vi "P2018 TB INCAR_Run Manual.vi"(7 "Comunicaciones":T7={"Flujo_1"="ASRL6::INSTR", "Brk1"=FALSE, "Flujo_2"="ASRL6::INSTR", "Brk2"=FALSE, "Flujo_3"="ASRL6::INSTR", "Brk3"=FALSE, "Flujo_4"="ASRL6::INSTR", "Brk4"=FALSE, "Eurothe"="ASRL6::INSTR", "Eurot"=FALSE, "Balanza"="ASRL6::INSTR", "Bal"=FALSE, "eValPos"="ASRL6::INSTR", "eVal"=FALSE, "flowbus"="ASRL6::INSTR", "fb"=FALSE}, 8 "error in (no error)":errorcluster) -> (0 "error out":errorcluster)   [LabVIEW 2013]
uses:
  Controles/P2022 Datos Control.ctl
  Controles/P2018 Com Control.ctl
  modbusEurotherm P116_485/P2018 Eurotherm Control.ctl
  modbusEurotherm P116_485/4xP116.ctl
  Controles/P2018 Bronkhorst Control.ctl
  serialBronkhorst/_s_TablaBronkhorst.ctl
  Controles/P2018 DisbalTB Control.ctl
  Controles/P2018 Arduino Control.ctl
  Controles/Data Type.ctl
  Display/Display_Command Control.ctl
  Controles/P2018 runManual Control.ctl
  File/File_Module Control.ctl
  Timing/Timing_Module Control.ctl
  modbusEurotherm P116_485/Eurotherm_Hardware_Module Control.ctl
  serialTermobDisbal/Multicard III_Hardware_Module Control.ctl
  Controles/Change Control.ctl
  P2022 TB INCAR GLOBALES.vi
panel:
  out "FLOWBUS_MassFlows":T1={"Dispositivos"=[["3", "NO", "M0000013", "Air", "10", "ln/mn", "0", "0"], ["4", "NO", "M0000014", "Air", "10", "ln/mn", "0", "0"], ["5", "NO", "M0000015", "Air", "10", "ln/mn", "0", "0"], ["6", "NO", "M0000016", "Air", "10", "ln/mn", "0", "0"], ["7", "NO", "M0000017", "Air", "10", "ln/mn", "0", "0"], ["8", "NO", "M0000018", "Air", "10", "ln/mn", "0", "0"]], "NuevosSP"=[["0", "NO", "M0000013", "Air", "1", "ln/mn", "0", "0"], ["0", "NO", "M0000014", "Air", "1", "ln/mn", "0", "0"], ["0", "NO", "M0000015", "Air", "1", "ln/mn", "0", "0"], ["0", "NO", "M0000016", "Air", "1", "ln/mn", "0", "0"], ["0", "NO", "M0000017", "Air", "1", "ln/mn", "0", "0"], ["0", "NO", "M0000018", "Air", "1", "ln/mn", "0", "0"]], "Nodes"=4, "Delay(s)"=0.075}
  out "Time Elapsed":bool
  out "ARDUINO":T3
  out "TIEMPO (m)":dbl
  out "DISBAL":T4 caption="tarjetaPresion"
  out "Fecha":string caption="asd"
  out "SERIAL_MassFlows":T1={"Dispositivos"=[["3", "NO", "M0000013", "Air", "10", "ln/mn", "0", "0"], ["4", "NO", "M0000014", "Air", "10", "ln/mn", "0", "0"], ["5", "NO", "M0000015", "Air", "10", "ln/mn", "0", "0"], ["6", "NO", "M0000016", "Air", "10", "ln/mn", "0", "0"], ["7", "NO", "M0000017", "Air", "10", "ln/mn", "0", "0"], ["8", "NO", "M0000018", "Air", "10", "ln/mn", "0", "0"]], "NuevosSP"=[["0", "NO", "M0000013", "Air", "1", "ln/mn", "0", "0"], ["0", "NO", "M0000014", "Air", "1", "ln/mn", "0", "0"], ["0", "NO", "M0000015", "Air", "1", "ln/mn", "0", "0"], ["0", "NO", "M0000016", "Air", "1", "ln/mn", "0", "0"], ["0", "NO", "M0000017", "Air", "1", "ln/mn", "0", "0"], ["0", "NO", "M0000018", "Air", "1", "ln/mn", "0", "0"]], "Nodes"=4, "Delay(s)"=0.075}
  out "EURO_P116":T5
  out "Time":string caption="asd"
  out "Date":string caption="asd"
  out "ERRORES_T":i32=5 caption="Elapsed Time (s)"
  out "errorT":bool
  out "DATOS":T8 {"fFSET4" format="%.2g"; "fFSET3" format="%.2g"; "fFSET2" format="%.2g"; "fFSET1" format="%.2g"; "fFLUJO4" format="%.2g"; "fFLUJO2" format="%.2g"; "fFLUJO1" format="%.2g"; "fFLUJO3" format="%.2g"; "T_EXTRA" format="%.2g"; "TSET_EXTRA" format="%.2g"; "T_CINTA" format="%.2g"; "TSET_CINTA" format="%.2g"; "sFSET4" format="%.2g"; "POSICION" format="%.2g"; "TEMP_SUP" format="%.2g"; "TSET_SUP" format="%.2g"; "PESO_TB" format="%.2g"; "TEMP_TB" format="%.2g"; "TEMP_INF" format="%.2g"; "sFSET3" format="%.2g"; "sFSET2" format="%.2g"; "sFSET1" format="%.2g"; "V_VAPOR" format="%.2g"; "sFLUJO4" format="%.2g"; "sFLUJO2" format="%.2g"; "sFLUJO1" format="%.2g"; "TSET_INF" format="%.2g"; "TIEMPO" format="%.2g"; "sFLUJO3" format="%.2g"}
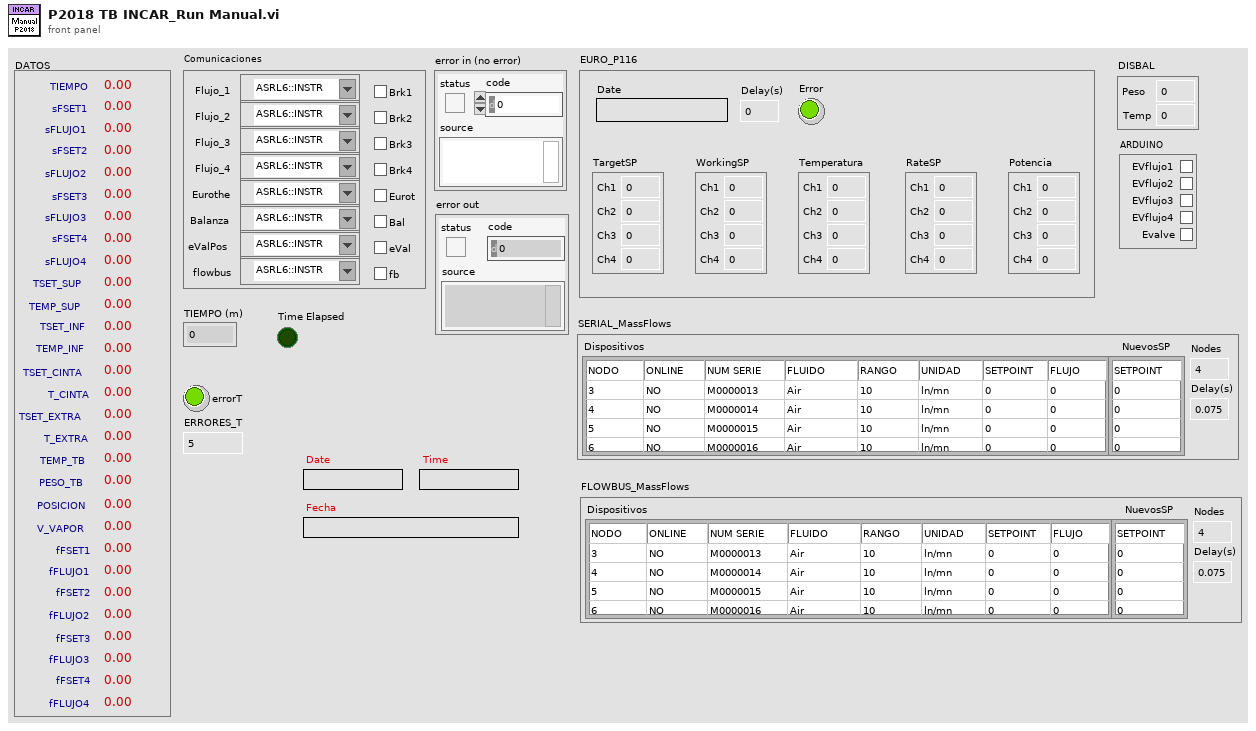
[diagram p1: front panel]
types:
  T1 = typedef "P2018 Bronkhorst Control.ctl" = cluster{"Dispositivos":T2, "NuevosSP":string[][], "Nodes":u32, "Delay(s)":dbl}
  T2 = typedef "_s_TablaBronkhorst.ctl" = string[][]
  T3 = typedef "P2018 Arduino Control.ctl" = cluster{"EVflujo1":bool, "EVflujo2":bool, "EVflujo3":bool, "EVflujo4":bool, "Evalve":bool}
  T4 = typedef "P2018 DisbalTB Control.ctl" = cluster{"Peso":dbl, "Temp":dbl}
  T5 = typedef "P2018 Eurotherm Control.ctl" = cluster{"TargetSP":T6, "WorkingSP":T6, "Temperatura":T6, "Error":bool, "Date":string, "Delay(s)":dbl, "RateSP":T6, "Potencia":T6}
  T6 = typedef "4xP116.ctl" = cluster{"Ch1":dbl, "Ch2":dbl, "Ch3":dbl, "Ch4":dbl}
  T7 = typedef "P2018 Com Control.ctl" = cluster{"Flujo_1":refnum<visa-resource-name>, "Brk1":bool, "Flujo_2":refnum<visa-resource-name>, "Brk2":bool, "Flujo_3":refnum<visa-resource-name>, "Brk3":bool, "Flujo_4":refnum<visa-resource-name>, "Brk4":bool, "Eurothe":refnum<visa-resource-name>, "Eurot":bool, "Balanza":refnum<visa-resource-name>, "Bal":bool, "eValPos":refnum<visa-resource-name>, "eVal":bool, "flowbus":refnum<visa-resource-name>, "fb":bool}
  T8 = typedef "P2022 Datos Control.ctl" = cluster{"TIEMPO":dbl, "sFSET1":dbl, "sFLUJO1":dbl, "sFSET2":dbl, "sFLUJO2":dbl, "sFSET3":dbl, "sFLUJO3":dbl, "sFSET4":dbl, "sFLUJO4":dbl, "TSET_SUP":dbl, "TEMP_SUP":dbl, "TSET_INF":dbl, "TEMP_INF":dbl, "TSET_CINTA":dbl, "T_CINTA":dbl, "TSET_EXTRA":dbl, "T_EXTRA":dbl, "TEMP_TB":dbl, "PESO_TB":dbl, "POSICION":dbl, "V_VAPOR":dbl, "fFSET1":dbl, "fFLUJO1":dbl, "fFSET2":dbl, "fFLUJO2":dbl, "fFSET3":dbl, "fFLUJO3":dbl, "fFSET4":dbl, "fFLUJO4":dbl}
  T9 = typedef "Data Type.ctl" = enum16{"Init FP", "En/Dis FP Ctls", "Update FP", "Upd Status", "Upd Seq"}
  T10 = typedef "Display_Command Control.ctl" = enum16{"Initialize", "Generate Event", "Shutdown"}
  T11 = typedef "P2018 runManual Control.ctl" = enum16{"INICIALIZAR", "READ BRONKHORST", "READ EUROTHERM", "READ DISBAL", "READ ARDUINO", "ESPERAR", "CAMBIOS", "GUARDAR", "FINALIZAR"}
  T12 = typedef "Timing_Module Control.ctl" = enum16{"Initialize Time", "Check Time"}
  T13 = typedef "File_Module Control.ctl" = enum16{"Initialize", "Save Head", "Save Data", "Shutdown"}
  T14 = typedef "Eurotherm_Hardware_Module Control.ctl" = enum16{"Initialize", "Write SP", "Read SP+PV", "Write Rate", "Set P", "Set I", "Set D", "Shutdown"}
  T15 = typedef "Multicard III_Hardware_Module Control.ctl" = enum16{"Initialize", "Cero", "Span", "Read ugr", "Read mgr", "Read A/D", "Read T", "Number readings", "Thermocouple type", "Status", "Shutdown"}
  T16 = typedef "Change Control.ctl" = enum16{"Default", "Continue", "Change Flows", "Change Valves", "Change Temp"}
  T17 = typedef "_f_TablaBronkhorst.ctl" = string[][]
  T18 = enum16{"Add 1", "Add 2", "Add 10", "Add 11", "Add 12", "Add 13"}[]
  T19 = cluster{"processVal":dbl, "targetSP":dbl, "workingSP":dbl, "workingOut":dbl}
  T20 = cluster{"[0]":dbl, "[1]":dbl, "[2]":dbl, "[3]":dbl}
  T21 = typedef "P2019 SetpointsFlows.ctl" = cluster{"SP1":dbl, "SP2":dbl, "SP3":dbl, "SP4":dbl}
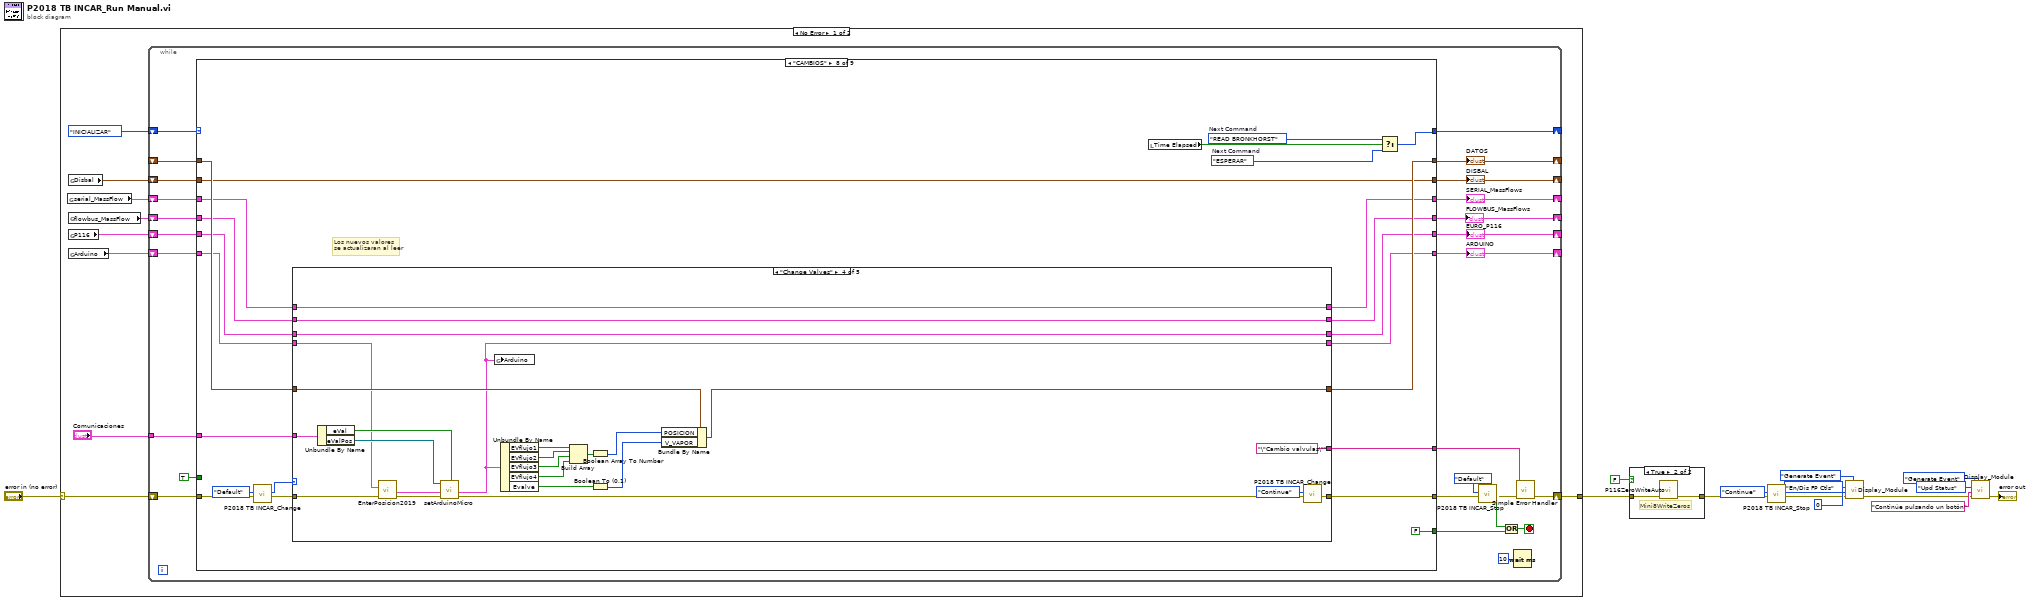
[diagram p0: block diagram]
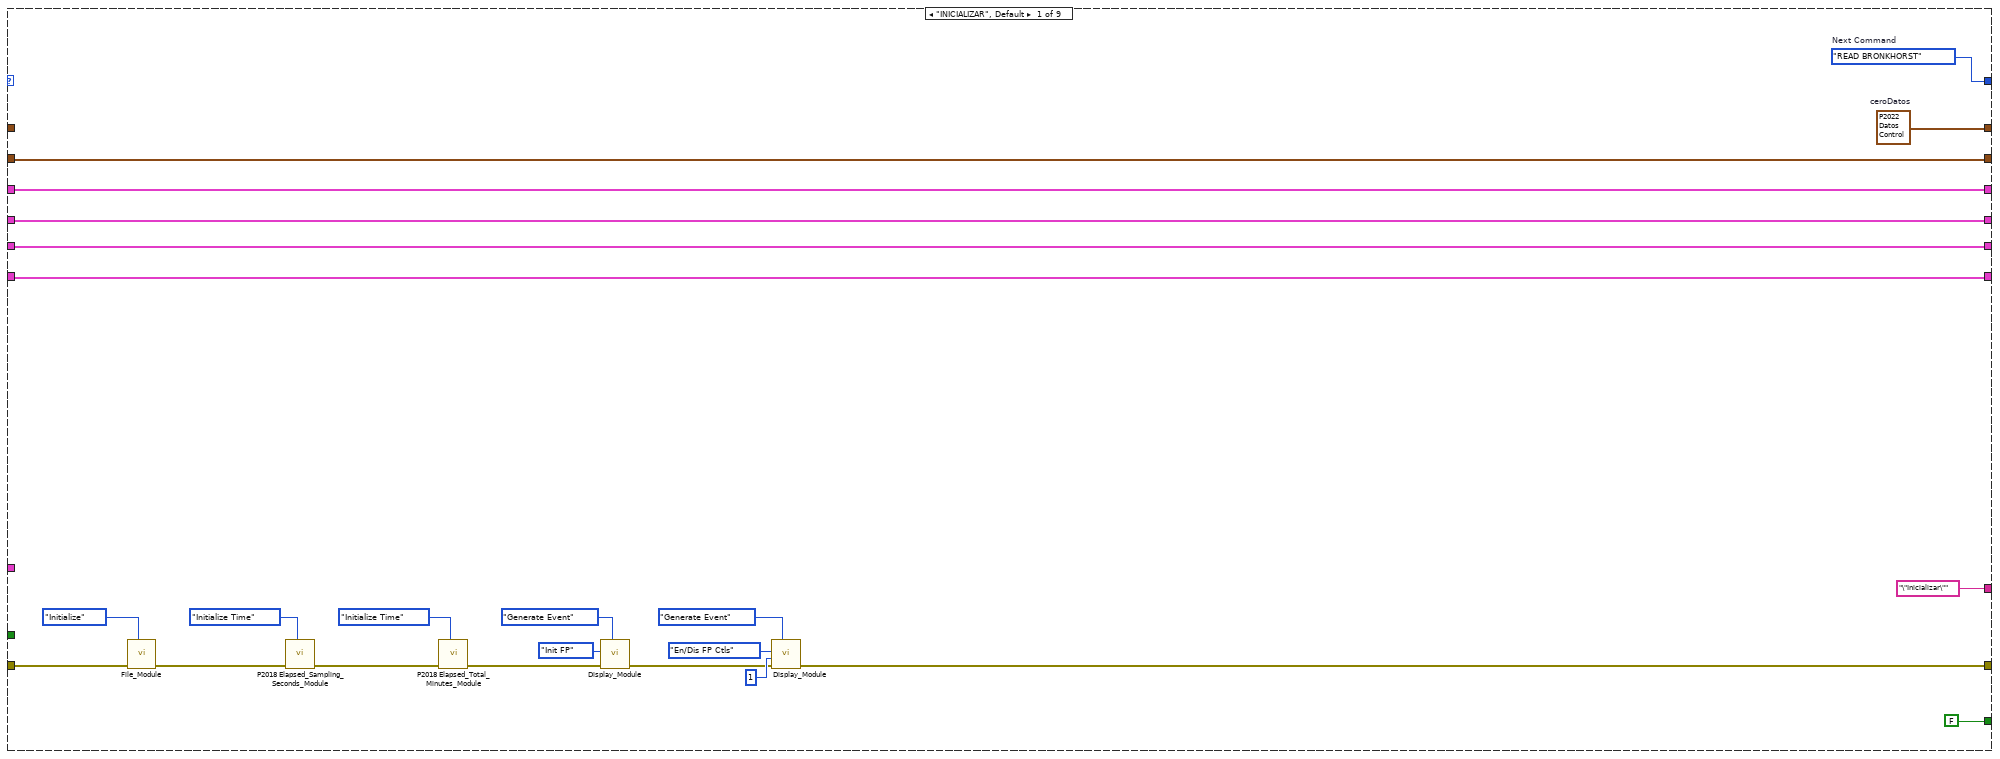
[diagram p3: hidden frame]
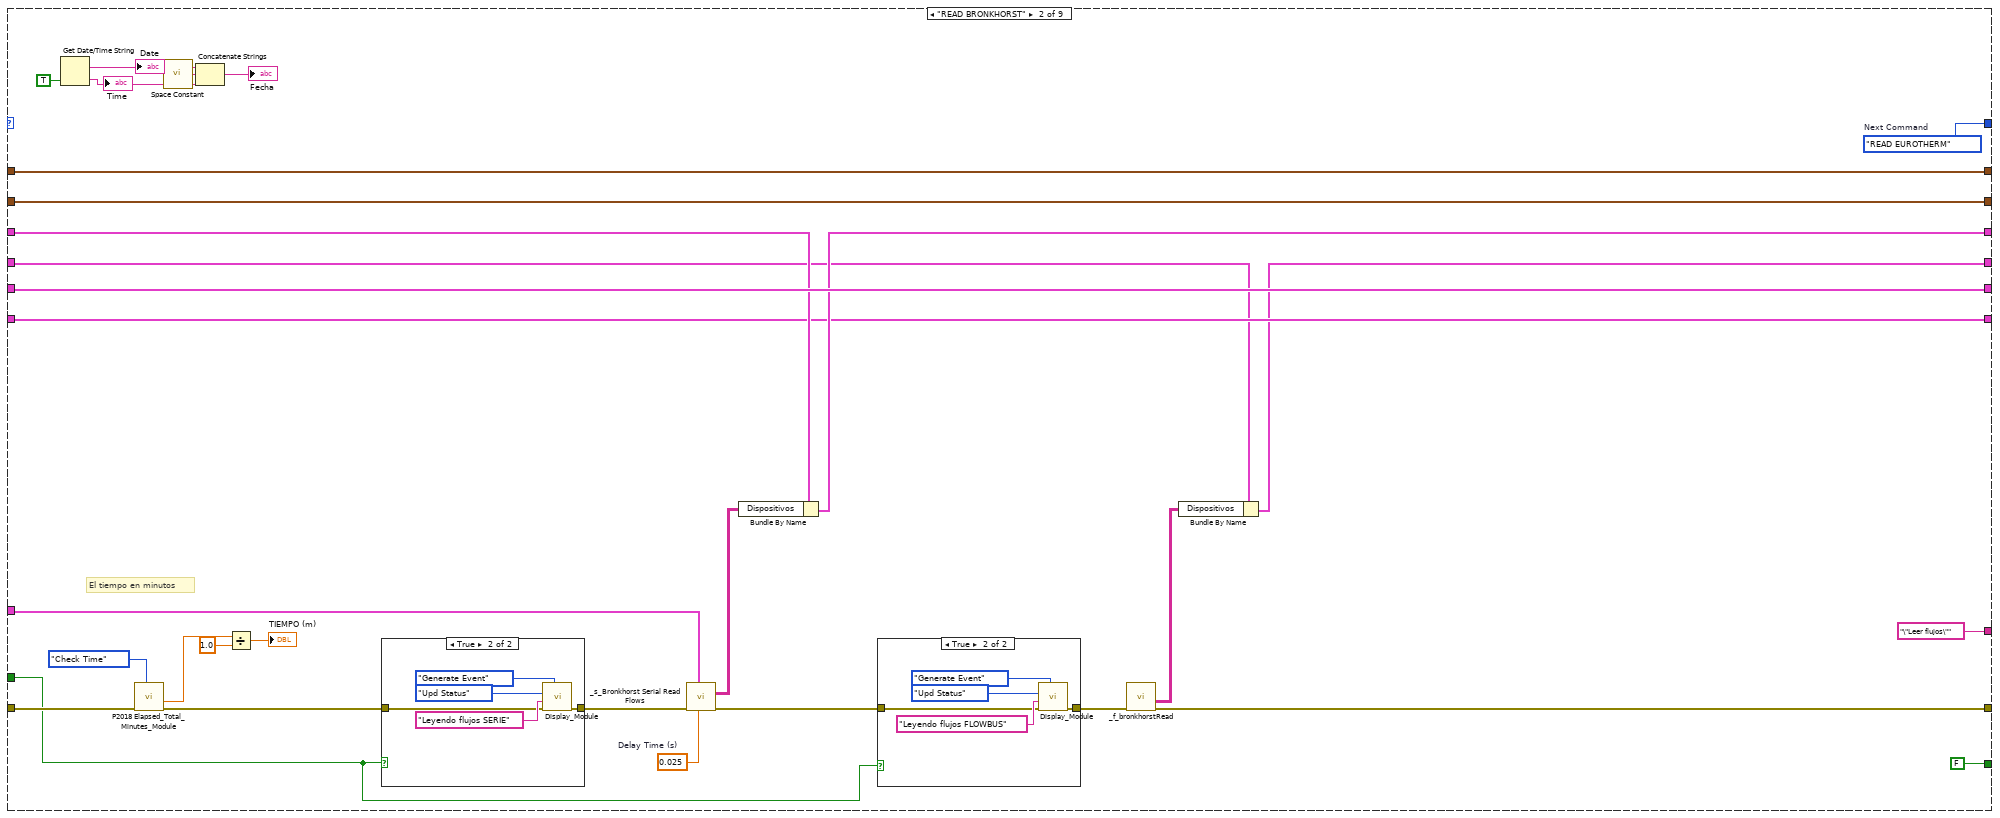
[diagram p4: hidden frame]
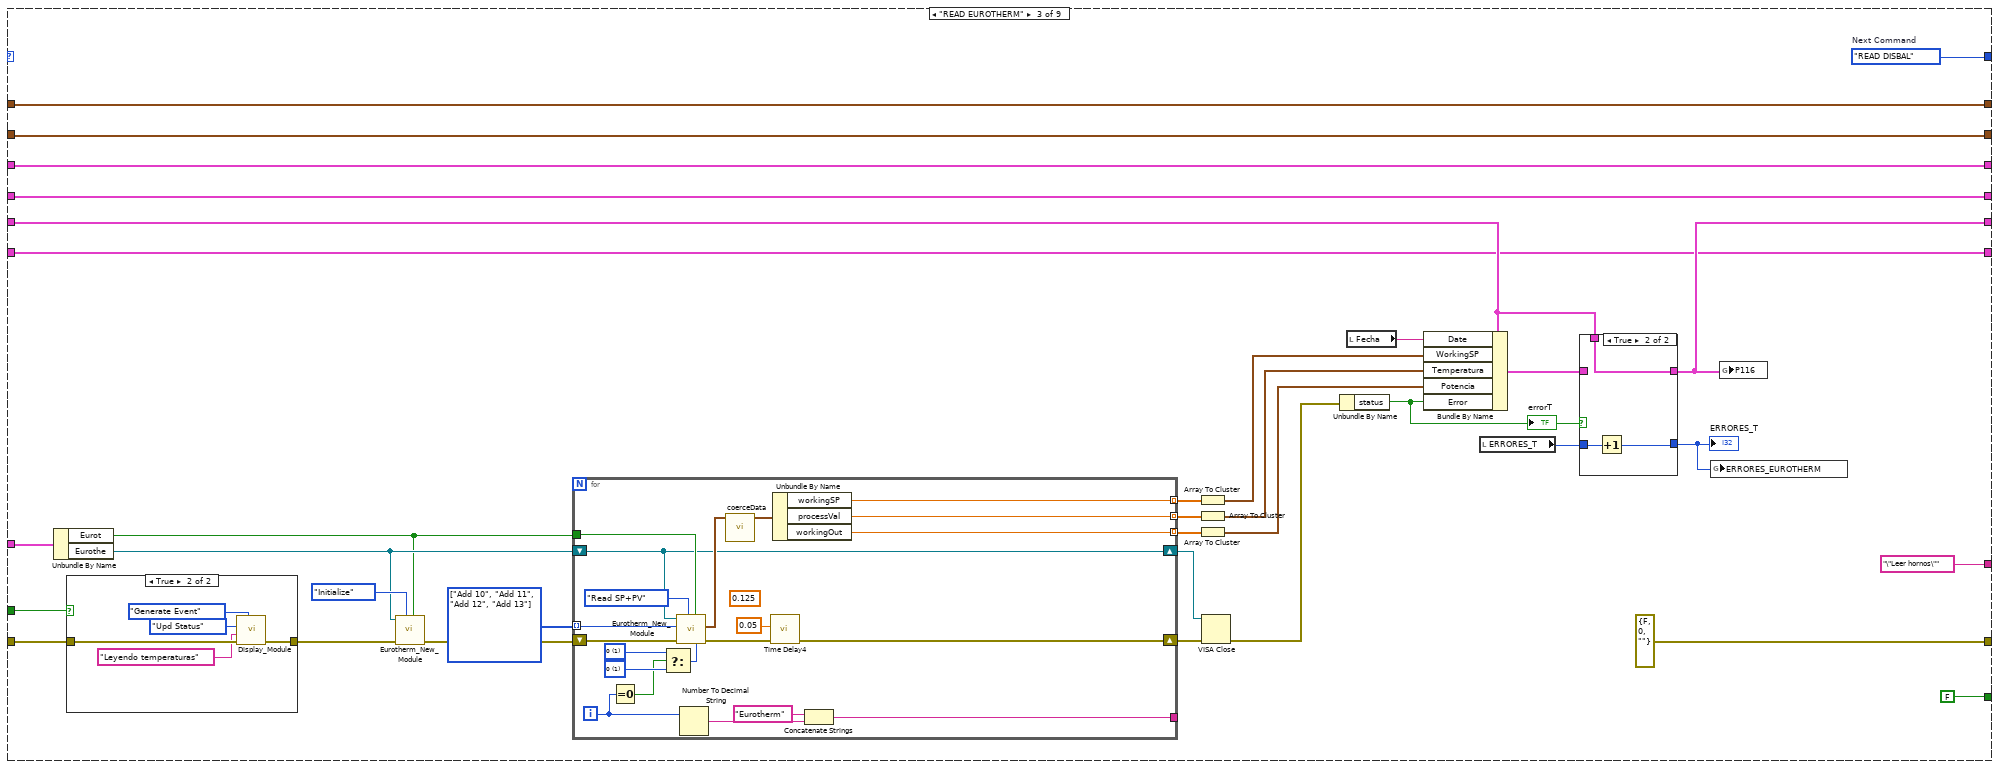
[diagram p7: hidden frame]
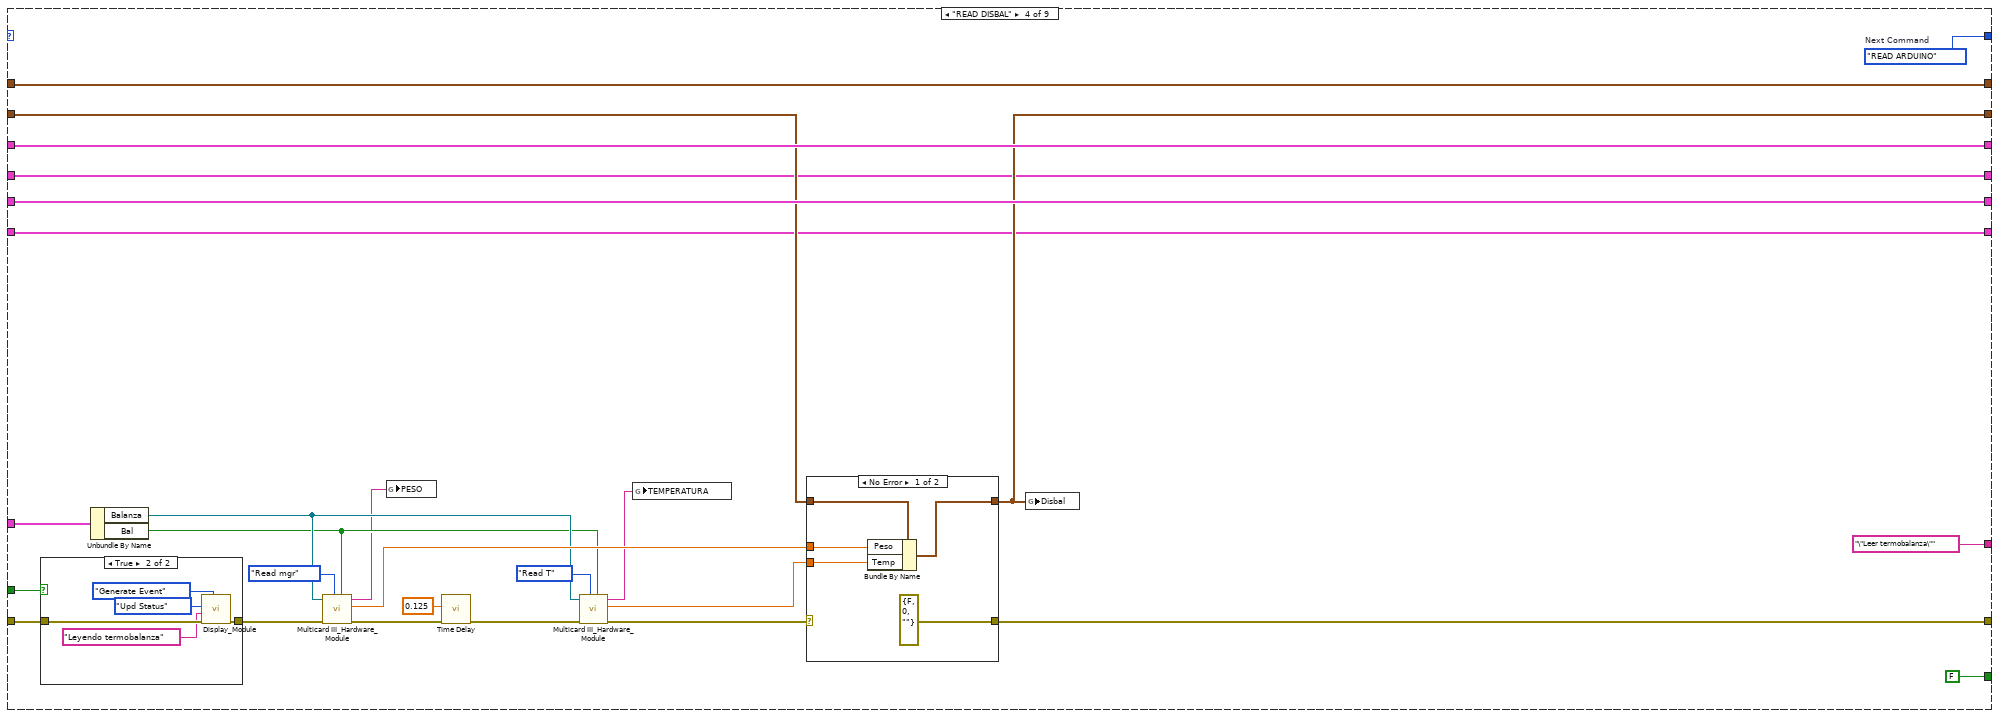
[diagram p10: hidden frame]
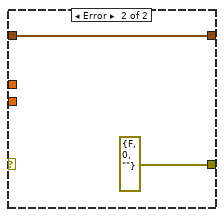
[diagram p12: hidden frame]
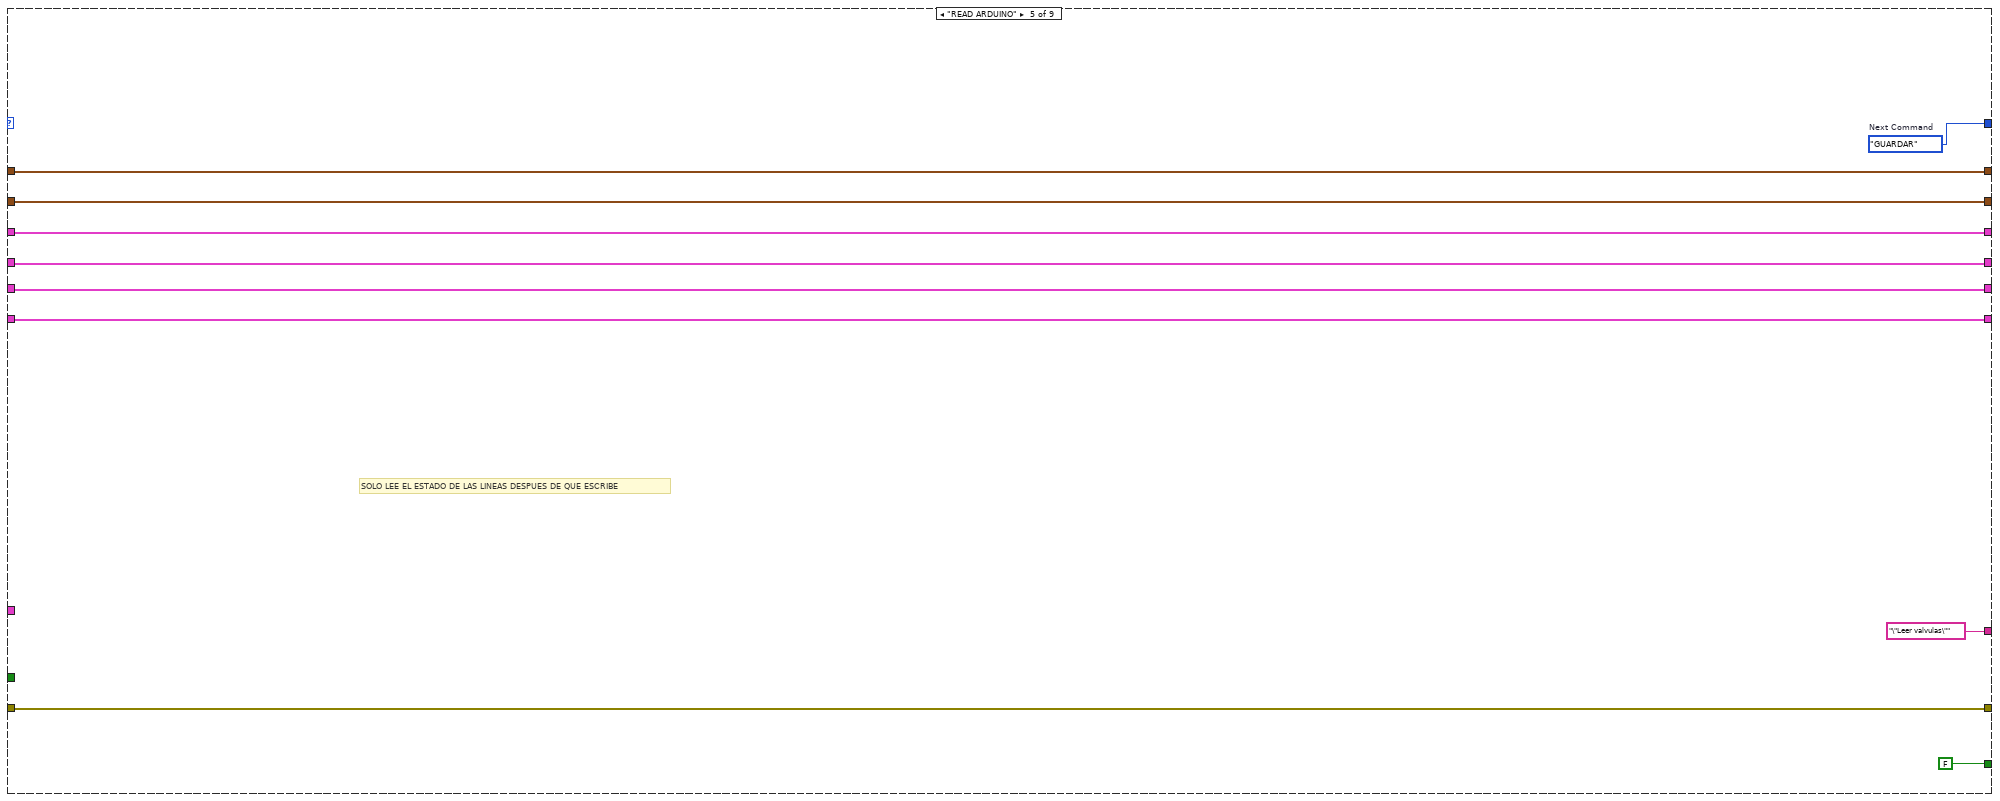
[diagram p13: hidden frame]
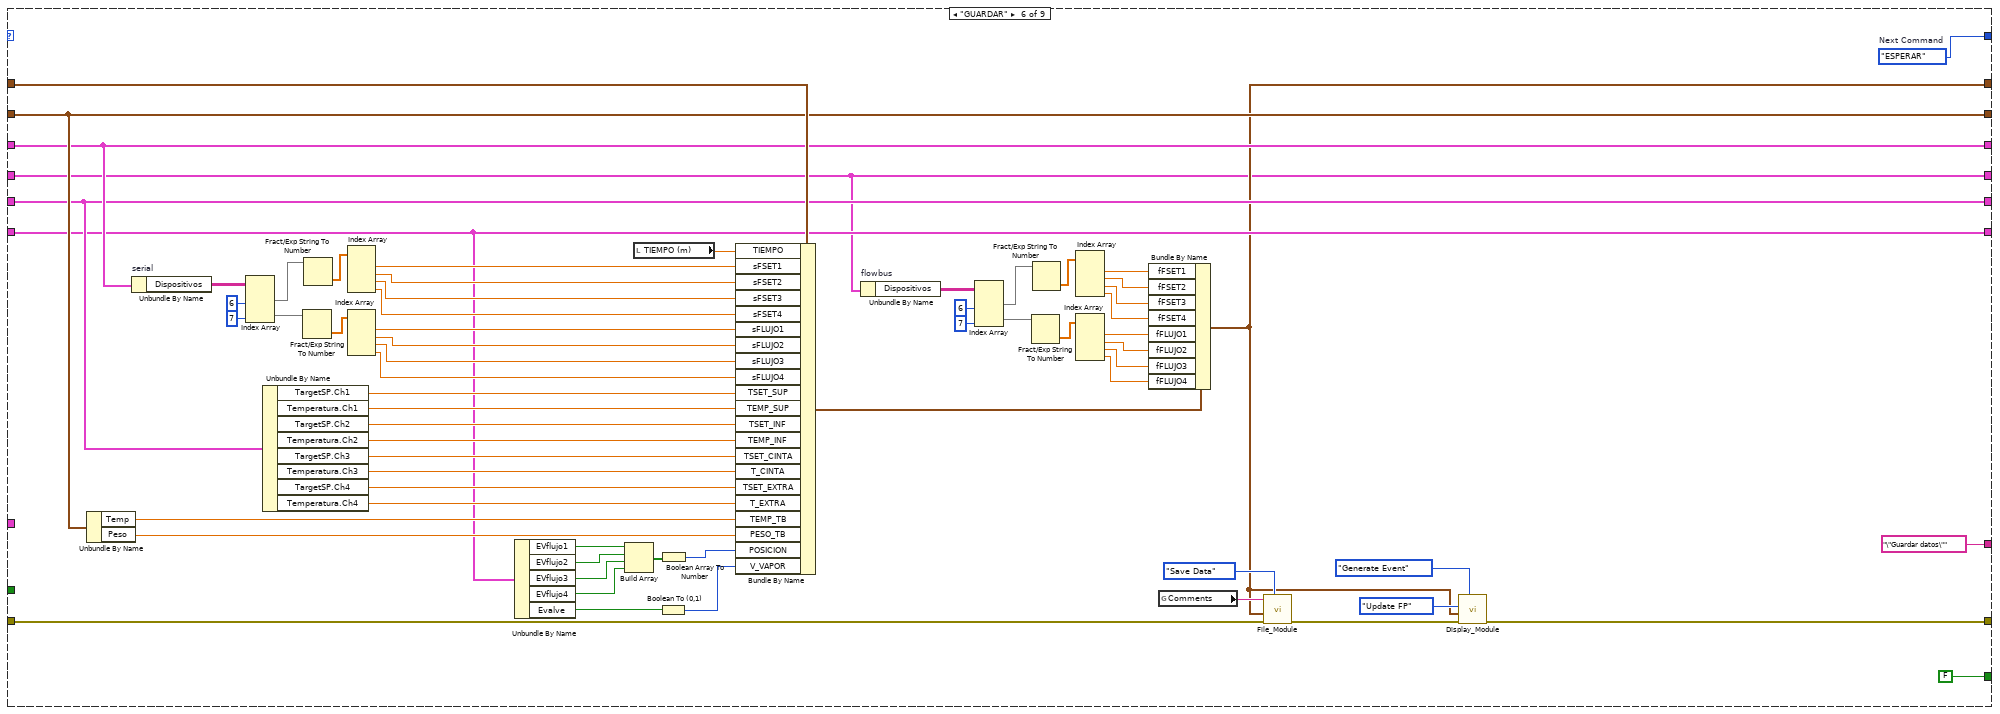
[diagram p14: hidden frame]
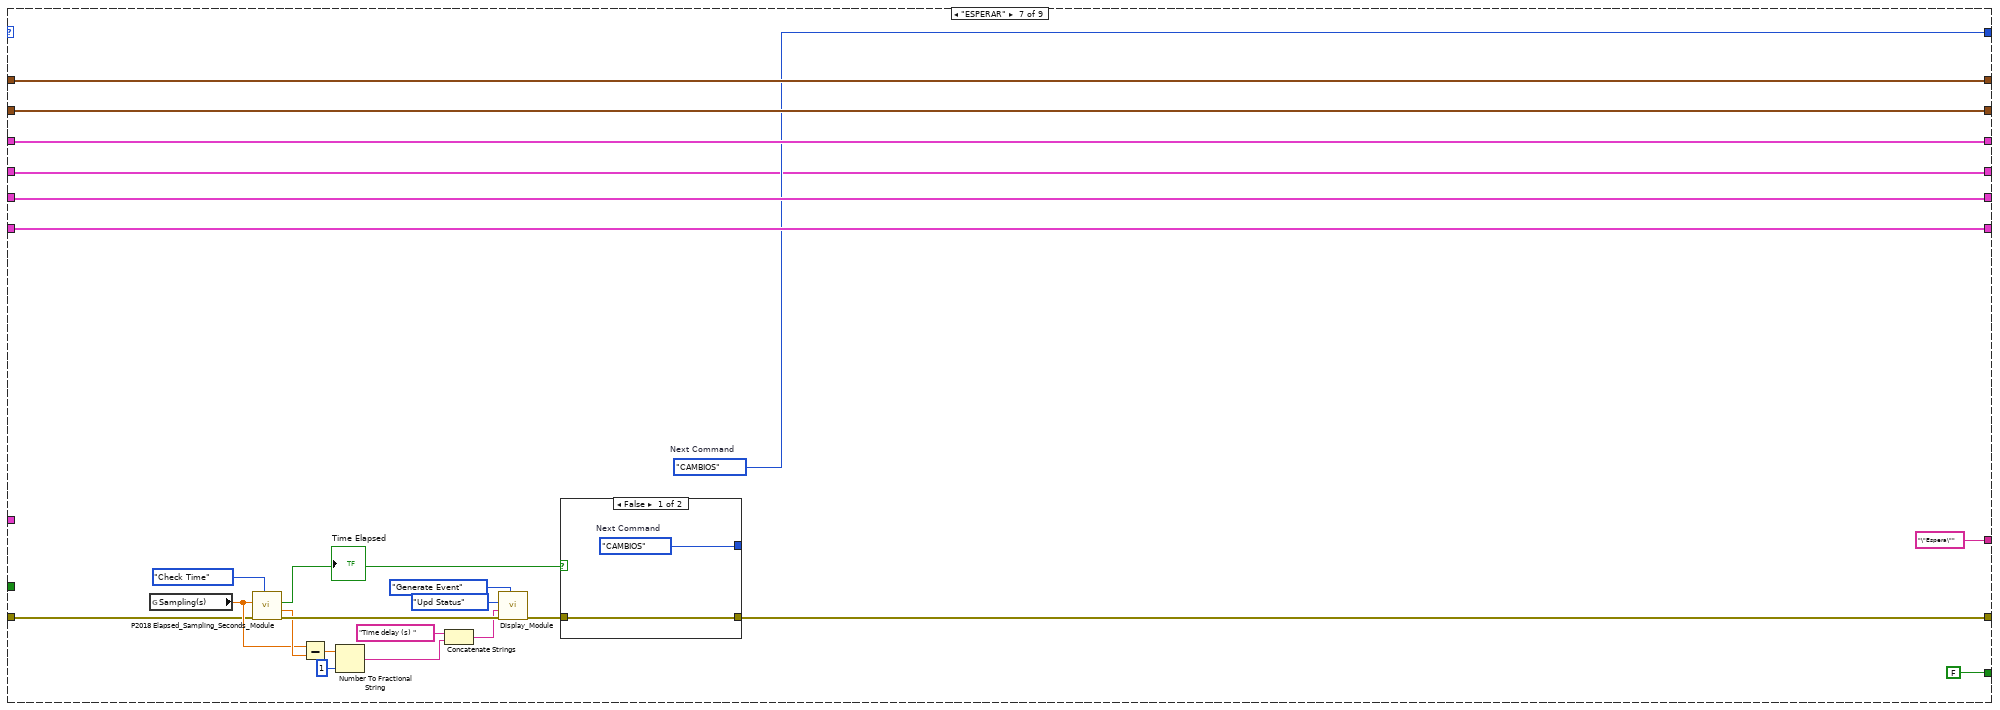
[diagram p15: hidden frame]
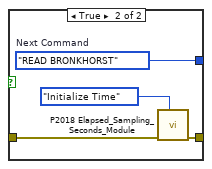
[diagram p16: hidden frame]
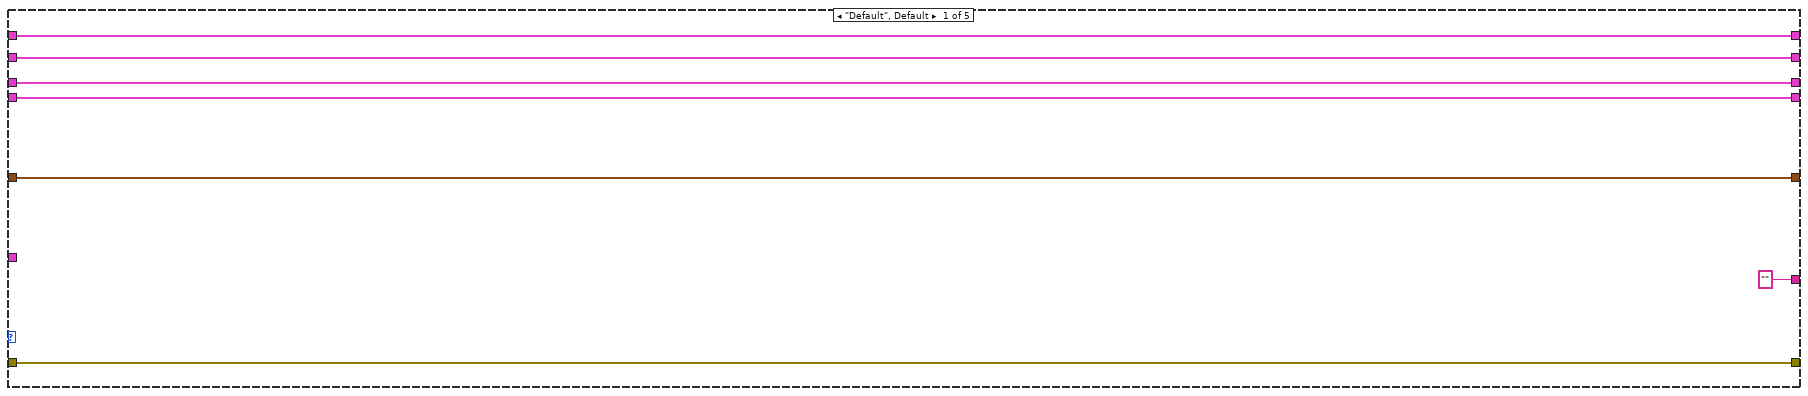
[diagram p17: hidden frame]
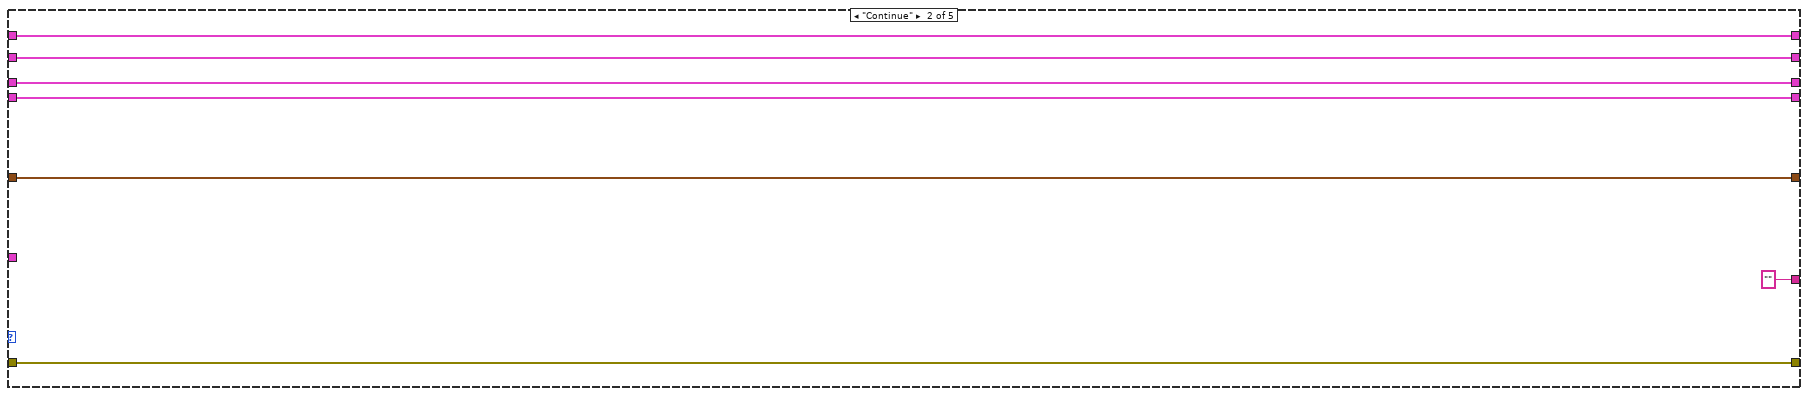
[diagram p18: hidden frame]
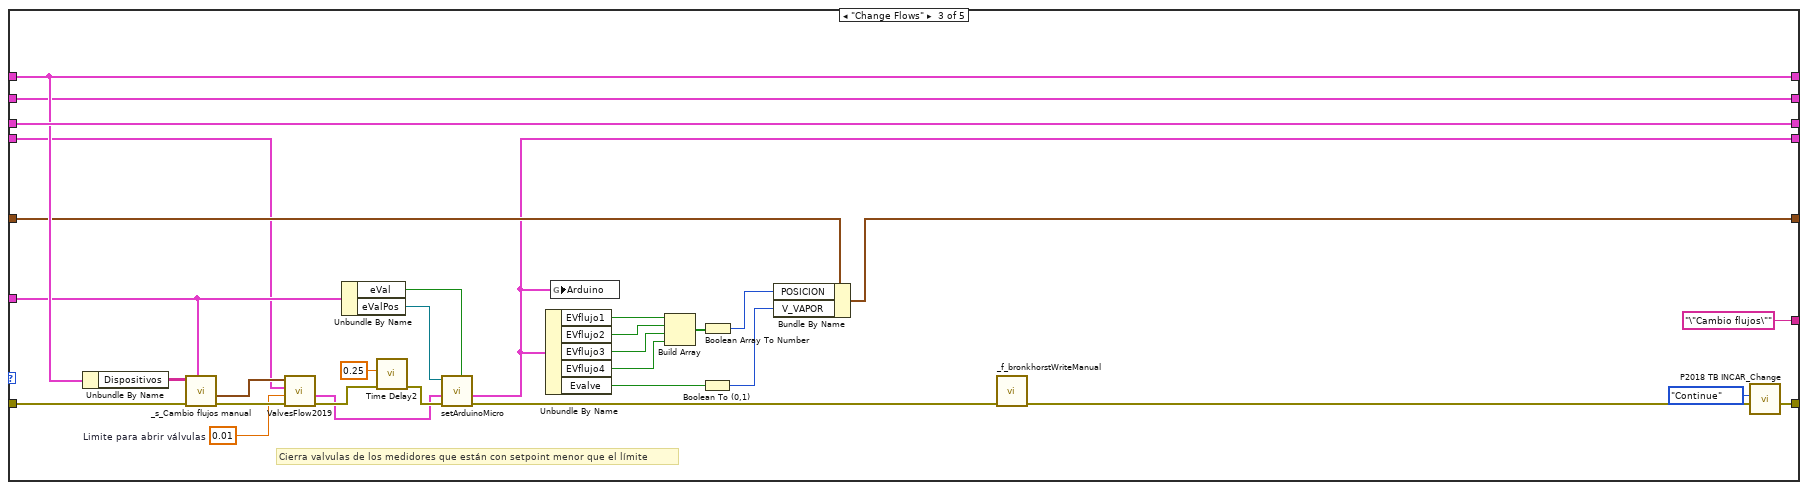
[diagram p19: hidden frame]
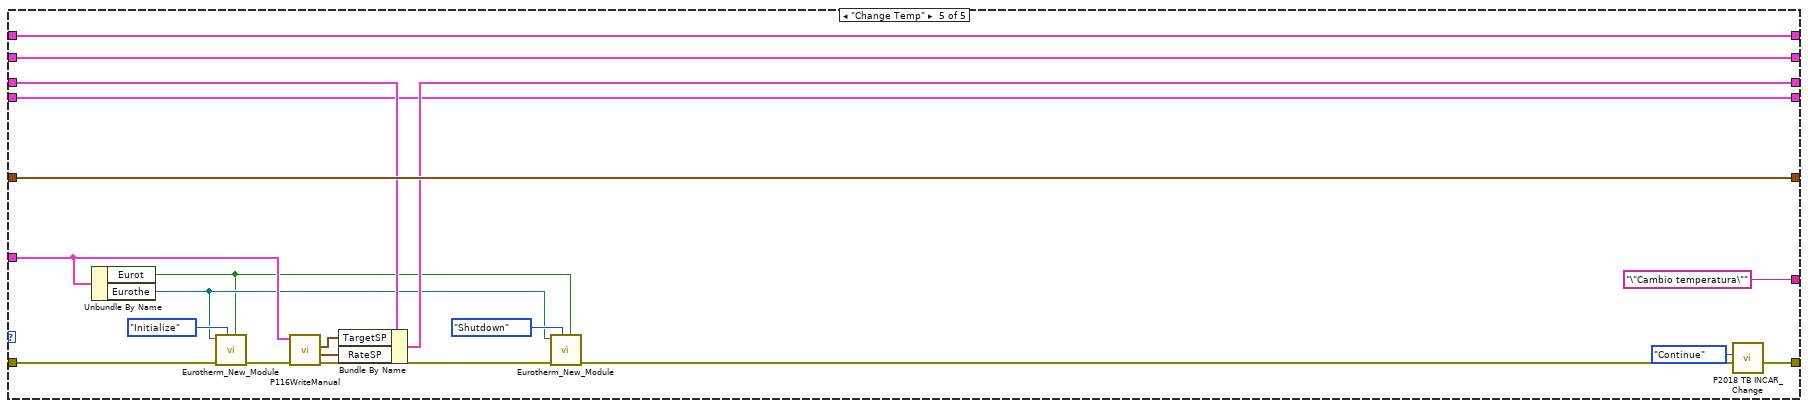
[diagram p20: hidden frame]
diagram:
  n1 = case shown="No Error" "error in (no error)" {
    selector: "error in (no error)" -> [w23 w453]
    tunnel: [w22 w453] -> w2
    frame No Error {
      n2 = global read "P2022 TB INCAR GLOBALES.vi" "serial_MassFlow"() -> (w18:T1)
      n3 = global read "P2022 TB INCAR GLOBALES.vi" "Disbal"() -> (w17:T4)
      n4 = global read "P2022 TB INCAR GLOBALES.vi" "flowbus_MassFlow"() -> (w15:T1)
      n5 = global read "P2022 TB INCAR GLOBALES.vi" "P116"() -> (w19:T5)
      n6 = global read "P2022 TB INCAR GLOBALES.vi" "Arduino"() -> (w16:T3)
      n7 = while {
        shift-right: [w42] -> _
        shift-left: P2018_runManual_Control."INICIALIZAR" ("Command") -> [w45]
        shift-right: [w36] -> w22
        shift-left: w23 -> [w46]
        shift-right: [w41] -> _
        shift-left: _ -> [w40]
        tunnel: "Comunicaciones" -> [w38]
        shift-right: [w30] -> _
        shift-left: w18 -> [w34]
        shift-right: [w32] -> _
        shift-left: w19 -> [w33]
        shift-right: [w29] -> _
        shift-left: w17 -> [w31]
        shift-right: [w27] -> _
        shift-left: w16 -> [w28]
        shift-right: [w24] -> _
        shift-left: w15 -> [w25]
        stop <- w48 stop-if-true
        n8 = case shown="\"CAMBIOS\"" w45 {
          tunnel: [FALSE FALSE FALSE FALSE FALSE FALSE FALSE FALSE TRUE] -> w47
          tunnel: w46 -> [w71 w91 w148 w207 w228 w298 w306 w350 w451]
          tunnel: [w69 w79 errorcluster {"status"=FALSE, "code"=0, "source"=""} ("error out") w204 w228 w292 w319 w347 w451] -> w44
          tunnel: [w65 w102 w147 w205 w230 w290 w300 w332 w449] -> w42
          tunnel: [w70 w82 w133 w190 w229 w233 w318 w344 w450] -> w41
          tunnel: w40 -> [_ w82 w133 w190 w229 w289 w318 w345 w450]
          tunnel: w38 -> [_ w92 w146 w202 _ _ _ w343 _]
          tunnel: ["\"Inicializar\"" ("error source (\" \")") "\"Leer flujos\"" ("error source (\" \")") "\"Leer hornos\"" ("error source (\" \")") "\"Leer termobalanza\"" ("error source (\" \")") "\"Leer valvulas\"" ("error source (\" \")") "\"Guardar datos\"" ("error source (\" \")") "\"Espera\"" ("error source (\" \")") w342 "\"Finalizar\"" ("error source (\" \")")] -> w35
          tunnel: [w53 w85 w121 w191 w226 w285 w303 w337 w446] -> w30
          tunnel: w34 -> [w53 w86 w121 w191 w226 w285 w303 w338 w446]
          tunnel: [w54 w98 w120 w192 w225 w277 w304 w339 w447] -> w32
          tunnel: w33 -> [w54 w98 w130 w192 w225 w277 w304 w340 w447]
          tunnel: w31 -> [w52 w83 w119 w189 w224 w288 w302 w341 w445]
          tunnel: [w52 w83 w119 w188 w224 w288 w302 w341 w445] -> w29
          tunnel: [w51 w81 w118 w187 w223 w252 w301 w335 w444] -> w27
          tunnel: w28 -> [w51 w81 w118 w187 w223 w252 w301 w336 w444]
          tunnel: TRUE -> [_ w73 w117 w185 _ _ _ _ _]
          tunnel: w25 -> [w50 w77 w116 w184 w222 w232 w299 w330 w443]
          tunnel: [w50 w76 w116 w184 w222 w232 w299 w329 w443] -> w24
          frame "INICIALIZAR", Default {
            w65 = P2018_runManual_Control."READ BRONKHORST"  # Next Command
            w70 = T8 {"TIEMPO"=0.0, "sFSET1"=0.0, "sFLUJO1"=0.0, "sFSET2"=0.0, "sFLUJO2"=0.0, "sFSET3"=0.0, "sFLUJO3"=0.0, "sFSET4"=0.0, "sFLUJO4"=0.0, "TSET_SUP"=0.0, "TEMP_SUP"=0.0, "TSET_INF"=0.0, "TEMP_INF"=0.0, "TSET_CINTA"=0.0, "T_CINTA"=0.0, "TSET_EXTRA"=0.0, "T_EXTRA"=0.0, "TEMP_TB"=0.0, "PESO_TB"=0.0, "POSICION"=0.0, "V_VAPOR"=0.0, "fFSET1"=0.0, "fFLUJO1"=0.0, "fFSET2"=0.0, "fFLUJO2"=0.0, "fFSET3"=0.0, "fFLUJO3"=0.0, "fFSET4"=0.0, "fFLUJO4"=0.0}  # ceroDatos
            n9 = call "File_Module.vi"("Command"=File_Module_Control."Initialize", "error in (no error)"=w71) -> ("error out"=w58:errorcluster)  [unwired: 8 in, 1 out]
            n10 = call "P2018 Elapsed_Sampling_Seconds_Module.vi"("Command"=Timing_Module_Control."Initialize Time", "error in (no error)"=w58) -> ("error out"=w60:errorcluster)  [unwired: 7 in, 2 out]
            n11 = call "P2018 Elapsed_Total_Minutes_Module.vi"("Command"=Timing_Module_Control."Initialize Time", "error in (no error)"=w60) -> ("error out"=w61:errorcluster)  [unwired: 7 in, 2 out]
            n12 = call "Display_Module.vi"("Command"=Display_Command_Control."Generate Event", "error in (no error)"=w61, "Data Type"=Data_Type."Init FP") -> ("error out"=w62:errorcluster)  [unwired: 8 in]
            n13 = call "Display_Module.vi"("Command"=Display_Command_Control."Generate Event", "error in (no error)"=w62, "Data"=1, "Data Type"=Data_Type."En/Dis FP Ctls") -> ("error out"=w69:errorcluster)  [unwired: 7 in]
          }
          frame "READ BRONKHORST" {
            w80 = 0.025  # Delay Time (s)
            w102 = P2018_runManual_Control."READ EUROTHERM"  # Next Command
            # "El tiempo en minutos"
            n14 = Get Date/Time String(want seconds? (F)=TRUE) -> (date string=w97:string, time string=w96:string)  [unwired: 2 in]
            "Time" <- w96
            "Date" <- w97
            n15 = call "P2018 Elapsed_Total_Minutes_Module.vi"("Command"=Timing_Module_Control."Check Time", "error in (no error)"=w91) -> ("error out"=w88:errorcluster, "Elapsed Out"=w90:dbl)  [unwired: 7 in, 1 out]
            n16 = call <vilib>:"Space Constant.vi"() -> ("String"=w94:string)
            n17 = Concatenate Strings(w97, w94, w96) -> (→"Fecha":string)
            n18 = Divide(x=w90, y=1.0) -> (x/y=→"TIEMPO (m)":dbl)
            n19 = case shown="True" w73 {
              tunnel: [w110 w112] -> w89
              tunnel: w88 -> [w110 w111]
              frame False {
              }
              frame True {
                n20 = call "Display_Module.vi"("Command"=Display_Command_Control."Generate Event", "error in (no error)"=w111, "Data"="Leyendo flujos SERIE", "Data Type"=Data_Type."Upd Status") -> ("error out"=w112:errorcluster)  [unwired: 7 in]
              }
            }
            n21 = call "_s_Bronkhorst Serial Read Flows.vi"("Delay Time (s)"=w80, "Comunicaciones"=w92, "error in (no error)"=w89) -> ("error out"=w75:errorcluster, "Dispositivos"=w84:T2)  [unwired: 7 in]
            n22 = Bundle By Name(cluster=w86, "Dispositivos"=w84) -> (w85:T1)
            n23 = case shown="True" w73 {
              tunnel: [w104 w106] -> w74
              tunnel: w75 -> [w104 w105]
              frame False {
              }
              frame True {
                n24 = call "Display_Module.vi"("Command"=Display_Command_Control."Generate Event", "error in (no error)"=w105, "Data"="Leyendo flujos FLOWBUS", "Data Type"=Data_Type."Upd Status") -> ("error out"=w106:errorcluster)  [unwired: 7 in]
              }
            }
            n25 = call "_f_bronkhorstRead.vi"("error in (no error)"=w74) -> ("error out"=w79:errorcluster, "Dispositivos"=w78:T17)  [unwired: 9 in]
            n26 = Bundle By Name(cluster=w77, "Dispositivos"=w78) -> (w76:T1)
          }
          frame "READ EUROTHERM" {
            w142 = T18 [enum."Add 10", enum."Add 11", enum."Add 12", enum."Add 13"] items=["Add 1", "Add 2", "Add 10", "Add 11", "Add 12", "Add 13"]
            w147 = P2018_runManual_Control."READ DISBAL"  # Next Command
            n27 = Unbundle By Name(w146) -> ("Eurot"=w139:bool, "Eurothe"=w140:refnum<visa-resource-name>)
            n28 = case shown="True" w117 {
              tunnel: w148 -> [w150 w153]
              tunnel: [w150 w151] -> w141
              frame False {
              }
              frame True {
                n29 = call "Display_Module.vi"("Command"=Display_Command_Control."Generate Event", "error in (no error)"=w153, "Data"="Leyendo temperaturas", "Data Type"=Data_Type."Upd Status") -> ("error out"=w151:errorcluster)  [unwired: 7 in]
              }
            }
            n30 = call "Eurotherm_New_Module.vi"("Eurotherm (T:Enable)"=w139, "Command"=Eurotherm_Hardware_Module_Control."Initialize", "error in (no error)"=w141, "VISA resource name"=w140) -> ("error out"=w143:errorcluster)  [unwired: 6 in, 1 out]
            n31 = for {
              tunnel: w142 -> [w175] mode=indexing
              tunnel: [w167] -> w136 mode=indexing
              tunnel: [w166] -> w135 mode=indexing
              shift-right: [w163] -> w137
              shift-left: w143 -> [w177]
              tunnel: w139 -> [w174]
              tunnel: [w179] -> _
              tunnel: [w165] -> w134 mode=indexing
              shift-right: [w164] -> w138
              shift-left: w140 -> [w164]
              i -> [w173]
              (unwired) 0.125 ("Delay Time (s)")
              w171 = u16 1 items=["0"=1, "1"=10, "2"=100] ("Decimales")
              w172 = u16 1 items=["0"=1, "1"=10, "2"=100] ("Decimales")
              n32 = Equal To 0?(x=w173) -> (x = 0?=w170:bool)
              n33 = Select(t=w172, s=w170, f=w171) -> (s? t:f=w169:u16)
              n34 = call "Eurotherm_New_Module.vi"("Decimales"=w169, "Eurotherm (T:Enable)"=w174, "Command"=Eurotherm_Hardware_Module_Control."Read SP+PV", "error in (no error)"=w177, "Address"=w175, "VISA resource name"=w164) -> ("error out"=w176:errorcluster, "Eurotherm"=w168:T19)  [unwired: 4 in]
              n35 = Number To Decimal String(number=w173) -> (decimal integer string=w180:string)  [unwired: 1 in]
              n36 = call "coerceData.vi"("Eurotherm"=w168) -> ("Eurotherm 2"=w161:T19)  [unwired: 10 in]
              n37 = call "Time Delay4"("error in (no error)"=w176, "Delay Time (s)"=0.05) -> ("error out"=w163:errorcluster)  [unwired: 9 in]
              n38 = Unbundle By Name(w161) -> ("workingSP"=w167:dbl, "processVal"=w166:dbl, "workingOut"=w165:dbl)
              n39 = Concatenate Strings("Eurotherm" ("error source (\" \")"), w180) -> (w179:string)
            }
            n40 = Array To Cluster(array=w136) -> (cluster=w128:T20)
            n41 = Array To Cluster(array=w135) -> (cluster=w127:T20)
            n42 = Array To Cluster(array=w134) -> (cluster=w126:T20)
            n43 = VISA Close(VISA resource name=w138, error in (no error)=w137) -> (error out=w125:errorcluster)
            n44 = Unbundle By Name(w125) -> ("status"=w132:bool)
            "errorT" <- w132
            n45 = local read "Fecha"() -> (w129:string)
            n46 = Bundle By Name(cluster=w130, "Date"=w129, "WorkingSP"=w128, "Temperatura"=w127, "Potencia"=w126, "Error"=w132) -> (w131:T5)
            n47 = local read "ERRORES_T"() -> (w123:i32)
            n48 = case shown="True" w132 {
              tunnel: w131 -> [w157 _]
              tunnel: [w157 w160] -> w120
              tunnel: w130 -> [_ w160]
              tunnel: w123 -> [w156 w159]
              tunnel: [w156 w158] -> w122
              frame False {
              }
              frame True {
                n49 = Increment(x=w159) -> (x+1=w158:i32)
              }
            }
            "ERRORES_T" <- w122
            n50 = global write "P2022 TB INCAR GLOBALES.vi" "ERRORES_EUROTHERM"(w122) -> ()
            n51 = global write "P2022 TB INCAR GLOBALES.vi" "P116"(w120) -> ()
          }
          frame "READ DISBAL" {
            w205 = P2018_runManual_Control."READ ARDUINO"  # Next Command
            n52 = case shown="True" w185 {
              tunnel: w207 -> [w209 w212]
              tunnel: [w209 w211] -> w206
              frame False {
              }
              frame True {
                n53 = call "Display_Module.vi"("Command"=Display_Command_Control."Generate Event", "error in (no error)"=w212, "Data"="Leyendo termobalanza", "Data Type"=Data_Type."Upd Status") -> ("error out"=w211:errorcluster)  [unwired: 7 in]
              }
            }
            n54 = Unbundle By Name(w202) -> ("Balanza"=w195:refnum<visa-resource-name>, "Bal"=w186:bool)
            n55 = call "Multicard III_Hardware_Module.vi"("Multicard (T:Enable)"=w186, "Command"=Multicard_III_Hardware_Module_Control."Read mgr", "error in (no error)"=w206, "VISA resource name"=w195) -> ("error out"=w197:errorcluster, "Output Value"=w203:dbl, "String"=w183:string)  [unwired: 4 in, 1 out]
            n56 = global write "P2022 TB INCAR GLOBALES.vi" "PESO"(w183) -> ()
            n57 = call "Time Delay"("error in (no error)"=w197, "Delay Time (s)"=0.125) -> ("error out"=w196:errorcluster)  [unwired: 9 in]
            n58 = call "Multicard III_Hardware_Module.vi"("Multicard (T:Enable)"=w186, "Command"=Multicard_III_Hardware_Module_Control."Read T", "error in (no error)"=w196, "VISA resource name"=w195) -> ("error out"=w199:errorcluster, "Output Value"=w198:dbl, "String"=w182:string)  [unwired: 4 in, 1 out]
            n59 = global write "P2022 TB INCAR GLOBALES.vi" "TEMPERATURA"(w182) -> ()
            n60 = case shown="No Error" w199 {
              tunnel: [errorcluster {"status"=FALSE, "code"=0, "source"=""} ("error out") errorcluster {"status"=FALSE, "code"=0, "source"=""} ("error out")] -> w204
              tunnel: w203 -> [w216 _]
              tunnel: w189 -> [w218 w220]
              tunnel: [w217 w220] -> w188
              tunnel: w198 -> [w215 _]
              frame No Error {
                n61 = Bundle By Name(cluster=w218, "Peso"=w216, "Temp"=w215) -> (w217:T4)
              }
              frame Error {
              }
            }
            n62 = global write "P2022 TB INCAR GLOBALES.vi" "Disbal"(w188) -> ()
          }
          frame "READ ARDUINO" {
            w230 = P2018_runManual_Control."GUARDAR"  # Next Command
            # "SOLO LEE EL ESTADO DE LAS LINEAS DESPUES DE QUE ESCRIBE"
          }
          frame "GUARDAR" {
            w290 = P2018_runManual_Control."ESPERAR"  # Next Command
            n63 = Unbundle By Name(w288) -> ("Temp"=w286:dbl, "Peso"=w287:dbl)
            n64 = Unbundle By Name "serial"(w285) -> ("Dispositivos"=w284:T2)
            n65 = Index Array(array=w284, index (col) #1=6 ("disabled index (col)"), index (col) #2=7 ("disabled index (col)")) -> (element #1=w265:string[], element #2=w266:string[])  [unwired: 2 in]
            n66 = Unbundle By Name(w277) -> ("TargetSP.Ch1"=w276:dbl, "Temperatura.Ch1"=w269:dbl, "TargetSP.Ch2"=w275:dbl, "Temperatura.Ch2"=w270:dbl, "TargetSP.Ch3"=w271:dbl, "Temperatura.Ch3"=w272:dbl, "TargetSP.Ch4"=w273:dbl, "Temperatura.Ch4"=w274:dbl)
            n67 = Fract/Exp String To Number(string=w266) -> (number=w281:dbl[])  [unwired: 3 in, 1 out]
            n68 = Fract/Exp String To Number(string=w265) -> (number=w264:dbl[])  [unwired: 3 in, 1 out]
            n69 = Index Array(array=w264) -> (element #1=w263:dbl, element #2=w262:dbl, element #3=w261:dbl, element #4=w260:dbl)  [unwired: 4 in]
            n70 = Index Array(array=w281) -> (element #1=w282:dbl, element #2=w280:dbl, element #3=w279:dbl, element #4=w278:dbl)  [unwired: 4 in]
            n71 = Unbundle By Name(w252) -> ("EVflujo1"=w257:bool, "EVflujo2"=w256:bool, "EVflujo3"=w255:bool, "EVflujo4"=w254:bool, "Evalve"=w258:bool)
            n72 = Build Array(w257, w256, w255, w254) -> (w253:bool[])
            n73 = local read "TIEMPO (m)"() -> (w268:dbl)
            n74 = Boolean To (0,1)(Boolean=w258) -> (0, 1=w251:i16)
            n75 = Boolean Array To Number(Boolean array=w253) -> (number=w250:u32)
            n76 = Bundle By Name(cluster=w289, "TIEMPO"=w268, "sFSET1"=w263, "sFSET2"=w262, "sFSET3"=w261, "sFSET4"=w260, "sFLUJO1"=w282, "sFLUJO2"=w280, "sFLUJO3"=w279, "sFLUJO4"=w278, "TSET_SUP"=w276, "TEMP_SUP"=w269, "TSET_INF"=w275, "TEMP_INF"=w270, "TSET_CINTA"=w271, "T_CINTA"=w272, "TSET_EXTRA"=w273, "T_EXTRA"=w274, "TEMP_TB"=w286, "PESO_TB"=w287, "POSICION"=w250, "V_VAPOR"=w251) -> (w234:T8)
            n77 = Unbundle By Name "flowbus"(w232) -> ("Dispositivos"=w243:T2)
            n78 = Index Array(array=w243, index (col) #1=6 ("disabled index (col)"), index (col) #2=7 ("disabled index (col)")) -> (element #1=w248:string[], element #2=w247:string[])  [unwired: 2 in]
            n79 = Fract/Exp String To Number(string=w247) -> (number=w245:dbl[])  [unwired: 3 in, 1 out]
            n80 = Fract/Exp String To Number(string=w248) -> (number=w249:dbl[])  [unwired: 3 in, 1 out]
            n81 = Index Array(array=w249) -> (element #1=w241:dbl, element #2=w240:dbl, element #3=w239:dbl, element #4=w238:dbl)  [unwired: 4 in]
            n82 = Index Array(array=w245) -> (element #1=w242:dbl, element #2=w237:dbl, element #3=w236:dbl, element #4=w235:dbl)  [unwired: 4 in]
            n83 = Bundle By Name(cluster=w234, "fFSET1"=w241, "fFSET2"=w240, "fFSET3"=w239, "fFSET4"=w238, "fFLUJO1"=w242, "fFLUJO2"=w237, "fFLUJO3"=w236, "fFLUJO4"=w235) -> (w233:T8)
            n84 = global read "P2022 TB INCAR GLOBALES.vi" "Comments"() -> (w259:string)
            n85 = call "File_Module.vi"("Command"=File_Module_Control."Save Data", "error in (no error)"=w298, "DATOS"=w233, "Comments"=w259) -> ("error out"=w293:errorcluster)  [unwired: 6 in, 1 out]
            n86 = call "Display_Module.vi"("Command"=Display_Command_Control."Generate Event", "error in (no error)"=w293, "Data"=w233, "Data Type"=Data_Type."Update FP") -> ("error out"=w292:errorcluster)  [unwired: 7 in]
          }
          frame "ESPERAR" {
            w300 = P2018_runManual_Control."CAMBIOS"  # Next Command
            n87 = global read "P2022 TB INCAR GLOBALES.vi" "Sampling(s)"() -> (w307:dbl)
            n88 = call "P2018 Elapsed_Sampling_Seconds_Module.vi"("Command"=Timing_Module_Control."Check Time", "error in (no error)"=w306, "Time In"=w307) -> ("error out"=w316:errorcluster, "Elapsed Out"=w313:dbl, "Time Elapsed"=w308:bool)  [unwired: 6 in]
            "Time Elapsed" <- w308
            n89 = Subtract(x=w307, y=w313) -> (x-y=w314:dbl)
            n90 = Number To Fractional String(number=w314, precision (6)=i16 1) -> (F-format string=w309:string)  [unwired: 2 in]
            n91 = Concatenate Strings("Time delay (s) ", w309) -> (w310:string)
            n92 = call "Display_Module.vi"("Command"=Display_Command_Control."Generate Event", "error in (no error)"=w316, "Data"=w310, "Data Type"=Data_Type."Upd Status") -> ("error out"=w315:errorcluster)  [unwired: 7 in]
            n93 = case shown="False" w308 {
              tunnel: [w323 w325] -> _
              tunnel: w315 -> [w324 w327]
              tunnel: [w324 w326] -> w319
              frame False {
                w323 = P2018_runManual_Control."CAMBIOS"  # Next Command
              }
              frame True {
                w325 = P2018_runManual_Control."READ BRONKHORST"  # Next Command
                n94 = call "P2018 Elapsed_Sampling_Seconds_Module.vi"("Command"=Timing_Module_Control."Initialize Time", "error in (no error)"=w327) -> ("error out"=w326:errorcluster)  [unwired: 7 in, 2 out]
              }
            }
          }
          frame "CAMBIOS" {
            w331 = P2018_runManual_Control."READ BRONKHORST"  # Next Command
            w333 = P2018_runManual_Control."ESPERAR"  # Next Command
            # "Los nuevos valores\nse actualizaran al leer"
            n95 = call "P2018 TB INCAR_Change.vi"("error in (no error)"=w350, "Change"=Change_Control."Default") -> ("error out"=w348:errorcluster, "Change?"=w349:T16)  [unwired: 8 in]
            n96 = case shown="\"Change Valves\"" w349 {
              tunnel: w348 -> [w358 w365 w395 w412 w431]
              tunnel: [w358 w365 w397 w422 w442] -> w347
              tunnel: w345 -> [w357 w364 w376 w420 w440]
              tunnel: [w357 w364 w375 w419 w440] -> w344
              tunnel: w343 -> [_ _ w377 w415 w428]
              tunnel: ["" ("error source (\" \")") "" ("error source (\" \")") "\"Cambio flujos\"" ("error source (\" \")") "\"Cambio valvulas\"" ("error source (\" \")") "\"Cambio temperatura\"" ("error source (\" \")")] -> w342
              tunnel: w340 -> [w355 w362 w393 w417 w436]
              tunnel: [w355 w362 w393 w417 w435] -> w339
              tunnel: w338 -> [w354 w361 w391 w416 w425]
              tunnel: [w354 w361 w391 w416 w425] -> w337
              tunnel: w336 -> [w353 w360 w374 w399 w424]
              tunnel: [w353 w360 w373 w400 w424] -> w335
              tunnel: w330 -> [w352 w359 w368 w398 w423]
              tunnel: [w352 w359 w368 w398 w423] -> w329
              frame "Default", Default {
              }
              frame "Continue" {
              }
              frame "Change Flows" {
                w388 = 0.01  # Limite para abrir válvulas
                # "Cierra valvulas de los medidores que están con setpoint menor que el límite"
                n97 = Unbundle By Name(w391) -> ("Dispositivos"=w392:T2)
                n98 = call "_s_Cambio flujos manual.vi"("Comunicaciones"=w377, "error in (no error)"=w395, "Dispositivos"=w392) -> ("error out"=w390:errorcluster, "Setpoints"=w389:T21)  [unwired: 7 in]
                n99 = call "ValvesFlow2019.vi"("error in (no error)"=w390, "Limite"=w388, "ESTADO in"=w374, "Setpoints"=w389) -> ("error out"=w371:errorcluster, "ESTADO out"=w369:T3)  [unwired: 4 in]
                n100 = Unbundle By Name(w377) -> ("eVal"=w386:bool, "eValPos"=w387:refnum<visa-resource-name>)
                n101 = call "Time Delay2"("error in (no error)"=w371, "Delay Time (s)"=0.25) -> ("error out"=w370:errorcluster)  [unwired: 9 in]
                n102 = call "setArduinoMicro.vi"("Enable"=w386, "error in"=w370, "ESTADO"=w369, "VISA resource name"=w387) -> ("error out"=w367:errorcluster, "ESTADO 2"=w373:T3)  [unwired: 6 in]
                n103 = Unbundle By Name(w373) -> ("EVflujo1"=w384:bool, "EVflujo2"=w383:bool, "EVflujo3"=w382:bool, "EVflujo4"=w381:bool, "Evalve"=w385:bool)
                n104 = global write "P2022 TB INCAR GLOBALES.vi" "Arduino"(w373) -> ()
                n105 = Build Array(w384, w383, w382, w381) -> (w380:bool[])
                n106 = Boolean To (0,1)(Boolean=w385) -> (0, 1=w378:i16)
                n107 = Boolean Array To Number(Boolean array=w380) -> (number=w379:u32)
                n108 = Bundle By Name(cluster=w376, "POSICION"=w379, "V_VAPOR"=w378) -> (w375:T8)
                n109 = call "_f_bronkhorstWriteManual.vi"("error in (no error)"=w367) -> ("error out"=w366:errorcluster)  [unwired: 9 in, 1 out]
                n110 = call "P2018 TB INCAR_Change.vi"("error in (no error)"=w366, "Change"=Change_Control."Continue") -> ("error out"=w397:errorcluster)  [unwired: 8 in, 1 out]
              }
              frame "Change Valves" {
                n111 = Unbundle By Name(w415) -> ("eVal"=w413:bool, "eValPos"=w414:refnum<visa-resource-name>)
                n112 = call "EnterPosicion2019.vi"("error in (no error)"=w412, "ESTADO in"=w399) -> ("error out"=w411:errorcluster, "ESTADO out"=w410:T3)  [unwired: 4 in, 2 out]
                n113 = call "setArduinoMicro.vi"("Enable"=w413, "error in"=w411, "ESTADO"=w410, "VISA resource name"=w414) -> ("error out"=w409:errorcluster, "ESTADO 2"=w400:T3)  [unwired: 6 in]
                n114 = global write "P2022 TB INCAR GLOBALES.vi" "Arduino"(w400) -> ()
                n115 = Unbundle By Name(w400) -> ("EVflujo1"=w407:bool, "EVflujo2"=w406:bool, "EVflujo3"=w405:bool, "EVflujo4"=w404:bool, "Evalve"=w408:bool)
                n116 = Build Array(w407, w406, w405, w404) -> (w403:bool[])
                n117 = Boolean To (0,1)(Boolean=w408) -> (0, 1=w401:i16)
                n118 = Boolean Array To Number(Boolean array=w403) -> (number=w402:u32)
                n119 = Bundle By Name(cluster=w420, "POSICION"=w402, "V_VAPOR"=w401) -> (w419:T8)
                n120 = call "P2018 TB INCAR_Change.vi"("error in (no error)"=w409, "Change"=Change_Control."Continue") -> ("error out"=w422:errorcluster)  [unwired: 8 in, 1 out]
              }
              frame "Change Temp" {
                n121 = Unbundle By Name(w428) -> ("Eurot"=w426:bool, "Eurothe"=w427:refnum<visa-resource-name>)
                n122 = call "Eurotherm_New_Module.vi"("Eurotherm (T:Enable)"=w426, "Command"=Eurotherm_Hardware_Module_Control."Initialize", "error in (no error)"=w431, "VISA resource name"=w427) -> ("error out"=w430:errorcluster)  [unwired: 6 in, 1 out]
                n123 = call "P116WriteManual.vi"("error in (no error)"=w430, "Comunicaciones"=w428) -> ("error out"=w432:errorcluster, "RateSP(C/min) 2"=w437:T6, "NuevoSP(C) 2"=w438:T6)  [unwired: 7 in]
                n124 = Bundle By Name(cluster=w436, "TargetSP"=w438, "RateSP"=w437) -> (w435:T5)
                n125 = call "Eurotherm_New_Module.vi"("Eurotherm (T:Enable)"=w426, "Command"=Eurotherm_Hardware_Module_Control."Shutdown", "error in (no error)"=w432, "VISA resource name"=w427) -> ("error out"=w429:errorcluster)  [unwired: 6 in, 1 out]
                n126 = call "P2018 TB INCAR_Change.vi"("error in (no error)"=w429, "Change"=Change_Control."Continue") -> ("error out"=w442:errorcluster)  [unwired: 8 in, 1 out]
              }
            }
            n127 = local read "Time Elapsed"() -> (w334:bool)
            n128 = Select(t=w331, s=w334, f=w333) -> (s? t:f=w332:T11)
          }
          frame "FINALIZAR" {
            w449 = P2018_runManual_Control."FINALIZAR"  # Next Command
          }
        }
        "DATOS" <- w41
        "SERIAL_MassFlows" <- w30
        "EURO_P116" <- w32
        "DISBAL" <- w29
        "ARDUINO" <- w27
        "FLOWBUS_MassFlows" <- w24
        n129 = call "P2018 TB INCAR_Stop.vi"("error in (no error)"=w44, "Stop"=enum16{"Continue", "Stop", "Default"}."Default") -> ("error out"=w37:errorcluster, "Stop?"=w43:bool)  [unwired: 8 in]
        n130 = Or(x=w43, y=w47) -> (x .or. y?=w48:bool)
        n131 = Wait (ms)(milliseconds to wait=u32 10) -> ()  [unwired: 1 out]
        n132 = call <vilib>:"Simple Error Handler.vi"("error source (\" \")"=w35, "error in (no error)"=w37) -> ("error out"=w36:errorcluster)  [unwired: 3 in, 4 out]
      }
    }
    frame Error {
    }
  }
  n133 = case shown="True" FALSE {
    tunnel: w2 -> [w454 w456]
    tunnel: [w454 w455] -> w1
    frame False {
    }
    frame True {
      # "Mini8WriteZeros"
      n134 = call "P116ZeroWriteAuto.vi"("error in (no error)"=w456) -> ("error out"=w455:errorcluster)  [unwired: 6 in, 4 out]
    }
  }
  n135 = call "P2018 TB INCAR_Stop.vi"("error in (no error)"=w1, "Stop"=enum16{"Continue", "Stop", "Default"}."Continue") -> ("error out"=w5:errorcluster)  [unwired: 8 in, 1 out]
  n136 = call "Display_Module.vi"("Command"=Display_Command_Control."Generate Event", "error in (no error)"=w5, "Data"=0, "Data Type"=Data_Type."En/Dis FP Ctls") -> ("error out"=w4:errorcluster)  [unwired: 7 in]
  n137 = call "Display_Module.vi"("Command"=Display_Command_Control."Generate Event", "error in (no error)"=w4, "Data"="Continúe pulsando un botón", "Data Type"=Data_Type."Upd Status") -> ("error out"=→"error out":errorcluster)  [unwired: 7 in]
